vi "setVertical.vi"(7 "Chn":string, 8 "error in (no error)":errorcluster, 9 "Dc Offset":dbl, 10 "Range [V]":dbl, 11 "ScopeNi in":refnum<class "ScopeNi.lvclass">) -> (0 "error out":errorcluster, 3 "ScopeNi out":refnum<class "ScopeNi.lvclass">)   [LabVIEW 2023, in "ScopeNi.lvclass"]
doc: "<b>Author:</b> Wolfgang\n<b>Description:</b> configure the vertical range of a channel"
uses:
  ScopeNi.lvclass
  ScopeNi.lvclass/ScopeNi.ctl
panel:
  out "Vertical:Vertical Range":dbl
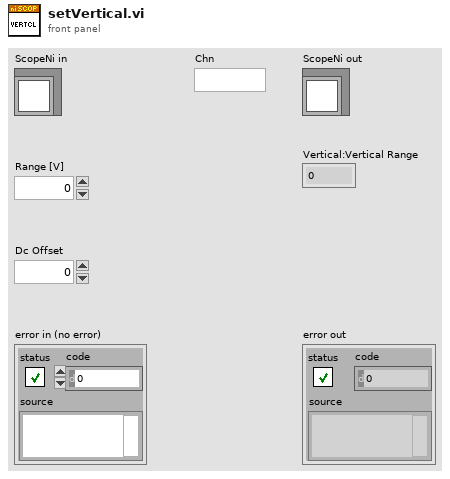
[diagram p1: front panel]
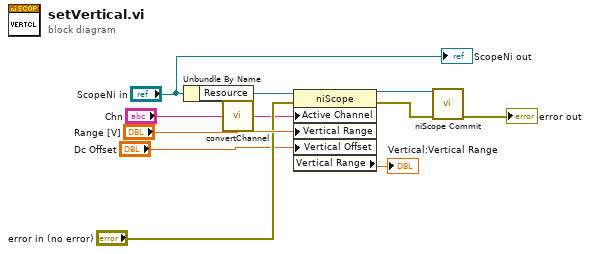
[diagram p0: block diagram]
diagram:
  n1 = Unbundle By Name("ScopeNi in") -> ("Resource"=w11:refnum<k15>)
  n2 = call "convertChannel.vi"("Chn in"="Chn") -> ("Chn out"=w5:string)
  n3 = property class="niScope"(reference=w11, error in="error in (no error)", "Active Channel"=w5, "Vertical Range"="Range [V]", "Vertical Offset"="Dc Offset") -> (reference out=w3:refnum<k15>, error out=w2:errorcluster, "Vertical Range"=→"Vertical:Vertical Range":dbl)
  n4 = call <instrlib>:"niScope Commit.vi"("instrument handle"=w3, "error in"=w2) -> ("error out"=→"error out":errorcluster)  [unwired: 12 in, 1 out]
  "ScopeNi out" <- "ScopeNi in"
